vi "GetConfig.vi"(8 "error in (no error)":errorcluster, 11 "ClientBase in":refnum<class "ClientBase.lvclass">) -> (0 "error out":errorcluster, 1 "Port":u16, 2 "Address":string, 3 "ClientBase out":refnum<class "ClientBase.lvclass">, 4 "ID":string)   [LabVIEW 2020, in "ClientBaseLib.lvlib" / "ClientBase.lvclass"]
uses:
  ClientBase.lvclass
  ClientBase.lvclass/ClientBase.ctl
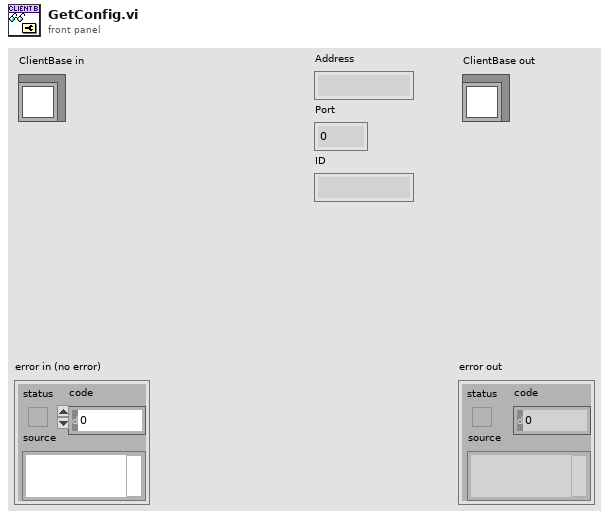
[diagram p1: front panel]
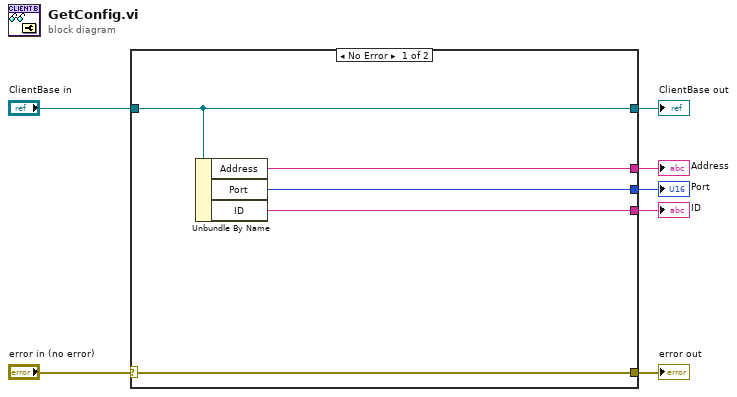
[diagram p0: block diagram]
diagram:
  n1 = case shown="No Error" "error in (no error)" {
    selector: "error in (no error)" -> [w12 w14]
    tunnel: [w12 w14] -> w6
    tunnel: [w11 w13] -> w4
    tunnel: "ClientBase in" -> [w11 w13]
    tunnel: [w10 _] -> w3
    tunnel: [w9 _] -> w2
    tunnel: [w8 _] -> w1
    frame No Error {
      n2 = Unbundle By Name(w11) -> ("Address"=w8:string, "Port"=w9:u16, "ID"=w10:string)
    }
    frame Error {
    }
  }
  "error out" <- w6
  "ClientBase out" <- w4
  "Address" <- w1
  "Port" <- w2
  "ID" <- w3
